vi "hms_rad.vi"(3 "True = hora":bool, 5 "Texto Graus":string) -> (2 "radianos":dbl format="%#.9f")   [LabVIEW 2012]
panel:
  out "before substring":string
  out "Erro":bool
  out "Segundos":dbl format="%.2f"
  out "Minutos":dbl
  out "Graus":dbl
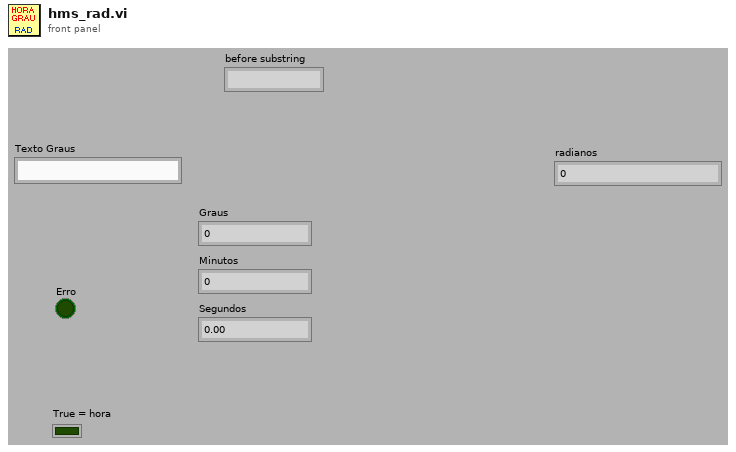
[diagram p1: front panel]
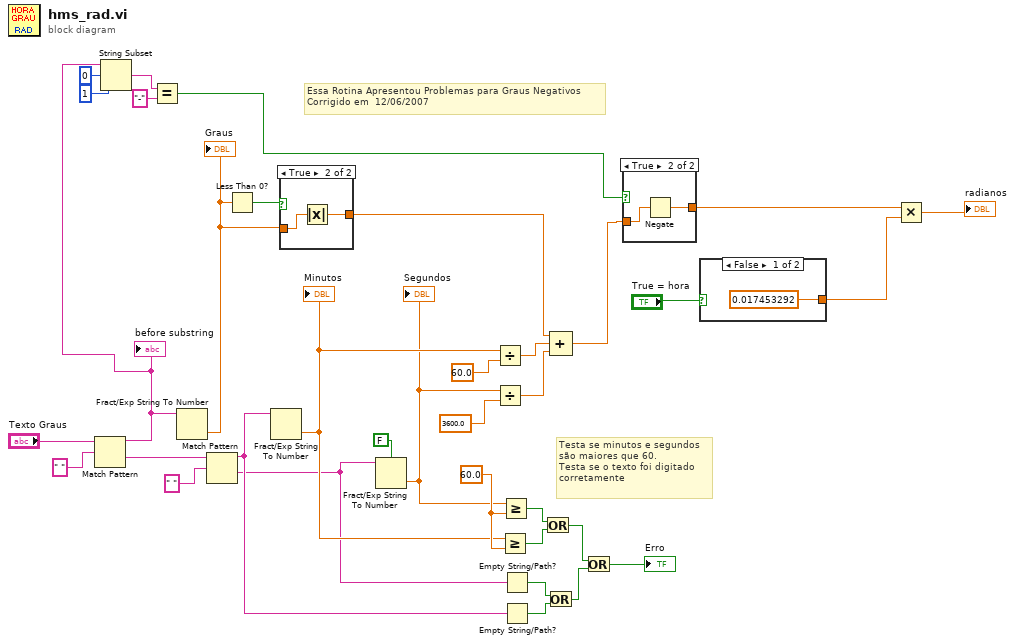
[diagram p0: block diagram]
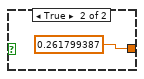
[diagram p2: hidden frame]
diagram:
  w26 = 60.0 ("x")
  # "Essa Rotina Apresentou Problemas para Graus Negativos\nCorrigido em  12/06/2007"
  # "Testa se minutos e segundos\nsão maiores que 60.\nTesta se o texto foi digitado\ncorretamente"
  n1 = Match Pattern(string="Texto Graus", regular expression=" ") -> (before substring=w10:string, after substring=w20:string)  [unwired: 1 in, 2 out]
  "before substring" <- w10
  n2 = String Subset(string=w10, offset (0)=0, length (rest)=1 ("length (rest)")) -> (substring=w7:string)
  n3 = Equal?(x=w7, y="-") -> (x = y?=w5:bool)
  n4 = Fract/Exp String To Number(string=w10) -> (number=w17:dbl)  [unwired: 3 in, 1 out]
  "Graus" <- w17
  n5 = Match Pattern(string=w20, regular expression=" ") -> (before substring=w19:string, after substring=w12:string)  [unwired: 1 in, 2 out]
  n6 = Less Than 0?(x=w17) -> (x < 0?=w13:bool)
  n7 = Fract/Exp String To Number(string=w19) -> (number=w18:dbl)  [unwired: 3 in, 1 out]
  "Minutos" <- w18
  n8 = case shown="True" w13 {
    tunnel: w17 -> [w36 w38]
    tunnel: [w36 w37] -> w16
    frame False {
    }
    frame True {
      n9 = Absolute Value(x=w38) -> (abs(x)=w37:dbl)
    }
  }
  n10 = Fract/Exp String To Number(use system decimal point (T)=FALSE, string=w12) -> (number=w11:dbl)  [unwired: 2 in, 1 out]
  "Segundos" <- w11
  n11 = Divide(x=w18, y=60.0) -> (x/y=w32:dbl)
  n12 = Divide(x=w11, y=3600.0) -> (x/y=w31:dbl)
  n13 = Greater Or Equal?(x=w18, y=w26) -> (x >= y?=w27:bool)
  n14 = Greater Or Equal?(x=w11, y=w26) -> (x >= y?=w28:bool)
  n15 = Empty String/Path?(string/path=w12) -> (empty?=w23:bool)
  n16 = Empty String/Path?(string/path=w19) -> (empty?=w22:bool)
  n17 = Or(x=w28, y=w27) -> (x .or. y?=w25:bool)
  n18 = Or(x=w23, y=w22) -> (x .or. y?=w21:bool)
  n19 = Compound Arithmetic op=ADD(w16, w32, w31) -> (w15:dbl)
  n20 = Or(x=w25, y=w21) -> (x .or. y?=→"Erro":bool)
  n21 = case shown="True" w5 {
    tunnel: w15 -> [w39 w41]
    tunnel: [w39 w40] -> w14
    frame False {
    }
    frame True {
      n22 = Negate(x=w41) -> (-x=w40:dbl)
    }
  }
  n23 = case shown="False" "True = hora" {
    tunnel: [0.017453292 ("y") 0.261799387 ("y")] -> w3
    frame False {
    }
    frame True {
    }
  }
  n24 = Multiply(x=w14, y=w3) -> (x*y=→"radianos":dbl)
